vi "Create Default Attributes.vi"(5 "Unique ID":string, 7 "Process Executive Ref":refnum<data-value>, 11 "Set Desired Station in":refnum<class "Set Desired Station.lvclass">) -> (3 "Set Desired Station out":refnum<class "Set Desired Station.lvclass">)   [LabVIEW 2019, in "Set Desired Station.lvclass"]
uses:
  <vilib>/gpm_packages/@cs/Car-wash/Source/Process Steps/Set Desired Station/Set Desired Station.lvclass
  <vilib>/gpm_packages/@cs/test-executive/Source/Test Executive/ITestExecutive/ITest Executive.lvclass
  8ebce20f-db5c-4b55-a670-2df1de1da25a.vi
  <vilib>/Utility/error.llb/Error Cluster From Error Code.vi
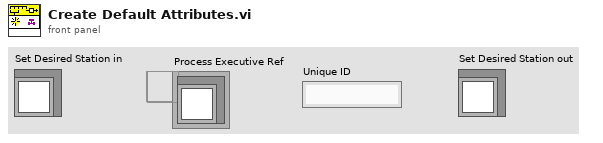
[diagram p1: front panel]
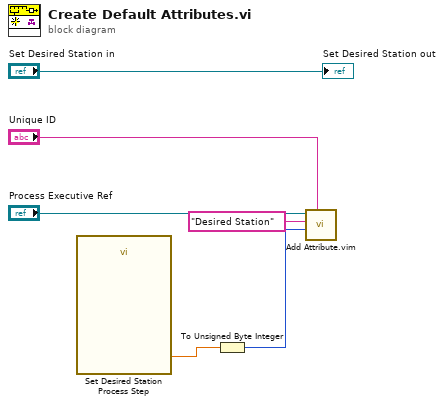
[diagram p0: block diagram]
diagram:
  n1 = call "Set Desired Station Process Step"() -> ("Station ID"=w2:dbl)  [unwired: 17 in, 2 out]
  n2 = To Unsigned Byte Integer(number=w2) -> (unsigned 8bit integer=w1:u8)
  n3 = call "Add Attribute.vim"("ID"="Unique ID", "Attribute"=w1, "Attribute Name"="Desired Station", "Test Executive Ref"="Process Executive Ref") -> ()  [unwired: 4 in, 4 out]
  "Set Desired Station out" <- "Set Desired Station in"
